vi "Contains Mouse.vi"(0 "FSM.Label":refnum<class "FSM.Label.lvclass">, 7 "Coords":T1) -> (4 "FSM.Label thru":refnum<class "FSM.Label.lvclass">, 8 "contains mouse":bool)   [LabVIEW 2020, in "FSM.Label.lvclass"]
uses:
  FSM.Label.lvclass
  <vilib>/Utility/miscctls.llb/LVPoint32TypeDef.ctl
  FSM.Label.lvclass/FSM.Label.ctl
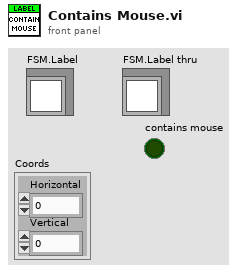
[diagram p1: front panel]
types:
  T1 = typedef "LVPoint32TypeDef.ctl" = cluster{"Horizontal":i32, "Vertical":i32}
  T2 = cluster{"left":i16, "top":i16, "right":i16, "bottom":i16}
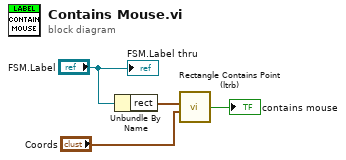
[diagram p0: block diagram]
diagram:
  n1 = Unbundle By Name("FSM.Label") -> ("rect"=w3:T2)
  n2 = call "Rectangle Contains Point (ltrb).vi"("Point"="Coords", "Rectangle"=w3) -> ("Contained?"=→"contains mouse":bool)  [unwired: 4 in]
  "FSM.Label thru" <- "FSM.Label"
